vi "flattenToString.vi"(8 "error in (no error)":errorcluster, 10 "Record":refnum<class "Record.lvclass">, 11 "Serializer.PlainText in":refnum<class "Serializer.PlainText.lvclass">) -> (0 "error out":errorcluster, 2 "Flattened String":string, 3 "Serializer.PlainText out":refnum<class "Serializer.PlainText.lvclass">)   [LabVIEW 2017, in "Serializer.Plug-in.lvlib" / "Serializer.PlainText.lvclass"]
uses:
  Serializer.PlainText.lvclass
  Record/Record.lvclass
  <vilib>/LabVIEW Open Source Project/OpenSerializer/Serializer.PlainText/Serializer.PlainText.lvclass
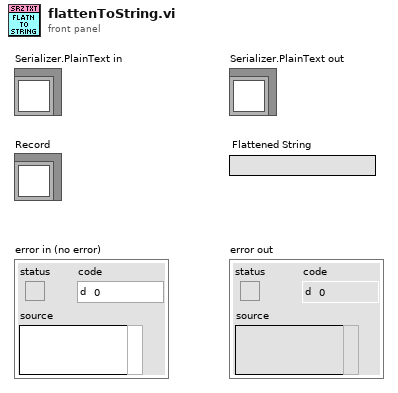
[diagram p1: front panel]
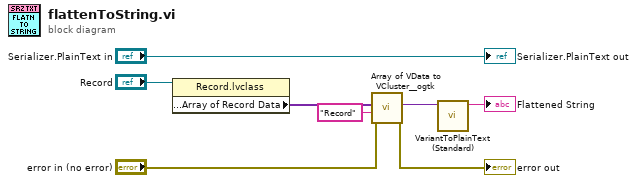
[diagram p0: block diagram]
diagram:
  n1 = property class="Record.lvclass"(reference="Record") -> ("Public API:Properties:Array of Record Data"=w8:variant[])  [unwired: 1 in, 2 out]
  n2 = call <userlib>:"Array of VData to VCluster__ogtk.vi"("error in (no error)"="error in (no error)", "Cluster Name"="Record", "Array"=w8) -> ("error out"=→"error out":errorcluster, "VCluster"=w7:variant)  [unwired: 7 in]
  n3 = call <vilib>:"VariantToPlainText (Standard).vi"("Variant-formatted Value"=w7) -> ("String-formatted Value"=→"Flattened String":string)  [unwired: 10 in]
  "Serializer.PlainText out" <- "Serializer.PlainText in"
